vi "Pull_Data_from_Server.vi"(3 "Path of File relative to EnFlo Data Root":path) -> (0 "error out":errorcluster, 1 "File String":string)   [LabVIEW 2011]
uses:
  Anemometry/Anemometry Sub Vis/Globals/Constants_global.vi
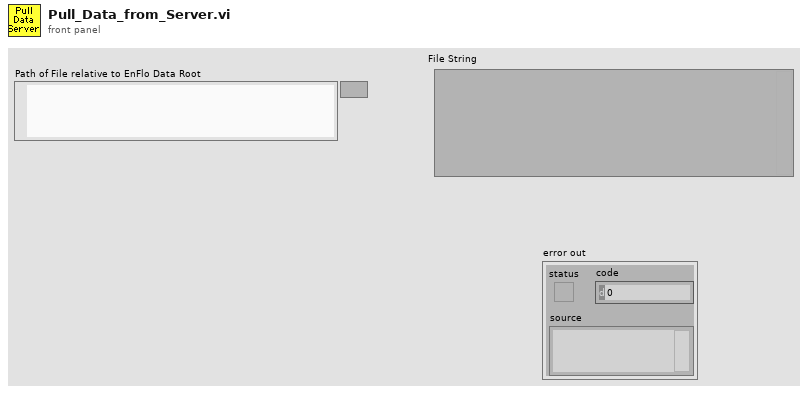
[diagram p1: front panel]
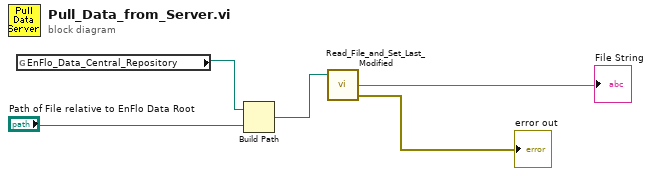
[diagram p0: block diagram]
diagram:
  n1 = global read "Constants_global.vi" "EnFlo_Data_Central_Repository"() -> (w5:path)
  n2 = Build Path(base path=w5, name or relative path="Path of File relative to EnFlo Data Root") -> (appended path=w3:path)
  n3 = call "Read_File_and_Set_Last_Modified.vi"("file path"=w3) -> ("error out"=→"error out":errorcluster, "string"=→"File String":string)  [unwired: 2 in, 1 out]
